vi "U64toRgba.vi"(11 "U64":u64) -> (3 "Rgba":T1)   [LabVIEW 2020, in "OpenLvVision_Image.lvlib" / "DataAccess.lvlib"]
doc: "Convert an number into an cluster"
uses:
  DataAccess.lvlib
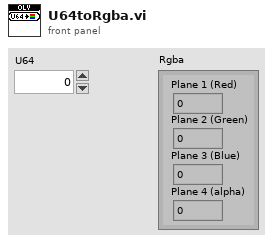
[diagram p1: front panel]
types:
  T1 = typedef "Color (U64)" = cluster{"Plane 3 (Blue)":u16, "Plane 2 (Green)":u16, "Plane 1 (Red)":u16, "Plane 4 (alpha)":u16}
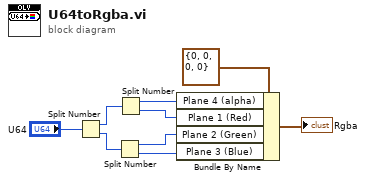
[diagram p0: block diagram]
diagram:
  n1 = Split Number(x="U64") -> (hi(x)=w8:u32, lo(x)=w7:u32)
  n2 = Split Number(x=w7) -> (hi(x)=w4:u16, lo(x)=w6:u16)
  n3 = Split Number(x=w8) -> (hi(x)=w5:u16, lo(x)=w3:u16)
  n4 = Bundle By Name(cluster=T1 {"Plane 3 (Blue)"=0, "Plane 2 (Green)"=0, "Plane 1 (Red)"=0, "Plane 4 (alpha)"=0} ("Rgba"), "Plane 4 (alpha)"=w5, "Plane 1 (Red)"=w3, "Plane 2 (Green)"=w4, "Plane 3 (Blue)"=w6) -> (→"Rgba":T1)
